vi "eepromtest.vi"() -> ()   [LabVIEW 2017]
uses:
  Traverse/ICNC/ICNC2.lvlib
panel:
  in  "unsigned 32bit integer 2":u32
  out "Value out 2":string
  out "Value out":string
  in  "String":string
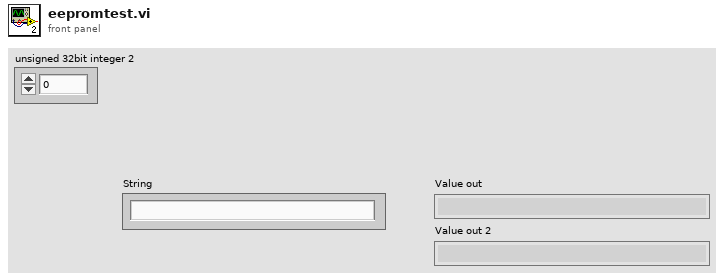
[diagram p1: front panel]
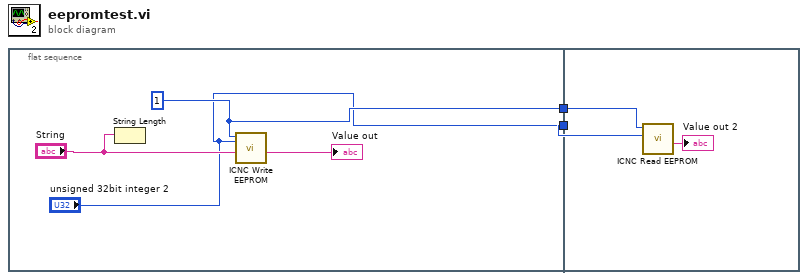
[diagram p0: block diagram]
diagram:
  n1 = flat-sequence {
    tunnel: ["unsigned 32bit integer 2"] -> w2
    tunnel: [w4] -> w1
    tunnel: w2 -> [w9]
    tunnel: w1 -> [w7]
    frame #0 {
      w4 = u32 1 ("StartAdress")
      n2 = String Length(string="String") -> ()  [unwired: 1 out]
      n3 = call <menus>:"ICNC Write EEPROM.vi"("Value"="String", "Length"="unsigned 32bit integer 2", "StartAdress"=w4) -> ("Value out"=→"Value out":string)  [unwired: 6 in, 2 out]
    }
    frame #1 {
      n4 = call <menus>:"ICNC Read EEPROM.vi"("Length"=w9, "StartAdress"=w7) -> ("Value out"=→"Value out 2":string)  [unwired: 7 in, 2 out]
    }
  }
